vi "MS SQL_InRFID_STN20.vi"(4 "[STATUS]":i32, 6 "RFID":string, 7 "OP10B_002_SLEEVE_PIN_SEAL_ASSY":T1, 8 "error in (no error)":errorcluster, 11 "Ref in":T2={"MS SQL Connection"=refnum, "UDL File"=path "", "Time"="", "DCODE"="", "WIP+1"=0, "MC No?"=0, "POKAYOKE?"=FALSE, "Expected Result"="", "Result [Status]"="", "Clock"=0.0, "RFID"="", "WIP Queue"=refnum, "TS Parameter"={"ProfitCenterCode"="", "LineCode"="", "WorkOrderNumber"="", "Model"="", "Model_with_Prefix"="", "VendorCode"="", "SetParameterDateCode"="", "PokaYoke"=0, "Target"=1, "Live_DateCode"="", "CustomerPartNumber"="", "Hand"="", "Ent_Stamp"=timestamp(0 s since 1904-01-01), "STS_CD"=0.0}, "Data_Queue"=[], "RFID Serial No."=""} {"TS Parameter"."Target" min=1 max=100000; "TS Parameter"."PokaYoke" min=0 max=1}) -> (0 "error out":errorcluster, 2 "Message":picture, 3 "Ref out":T2={"MS SQL Connection"=refnum, "UDL File"=path "", "Time"="", "DCODE"="", "WIP+1"=0, "MC No?"=0, "POKAYOKE?"=FALSE, "Expected Result"="", "Result [Status]"="", "Clock"=0.0, "RFID"="", "WIP Queue"=refnum, "TS Parameter"={"ProfitCenterCode"="", "LineCode"="", "WorkOrderNumber"="", "Model"="", "Model_with_Prefix"="", "VendorCode"="", "SetParameterDateCode"="", "PokaYoke"=0, "Target"=1, "Live_DateCode"="", "CustomerPartNumber"="", "Hand"="", "Ent_Stamp"=timestamp(0 s since 1904-01-01), "STS_CD"=0.0}, "Data_Queue"=[], "RFID Serial No."=""} {"TS Parameter"."Target" min=1 max=100000; "TS Parameter"."PokaYoke" min=0 max=1})   [LabVIEW 2020]
uses:
  Controls/TD SQL.ctl
  <vilib>/addons/database/Connection.llb/Conn ObjectReference.ctl
  Controls/WIP_State.ctl
  Controls/TS_Parameter.ctl
  Controls/OP10B_DataCluster.ctl
  <vilib>/addons/database/NI_Database_API.lvlib
panel:
  out "Query":string
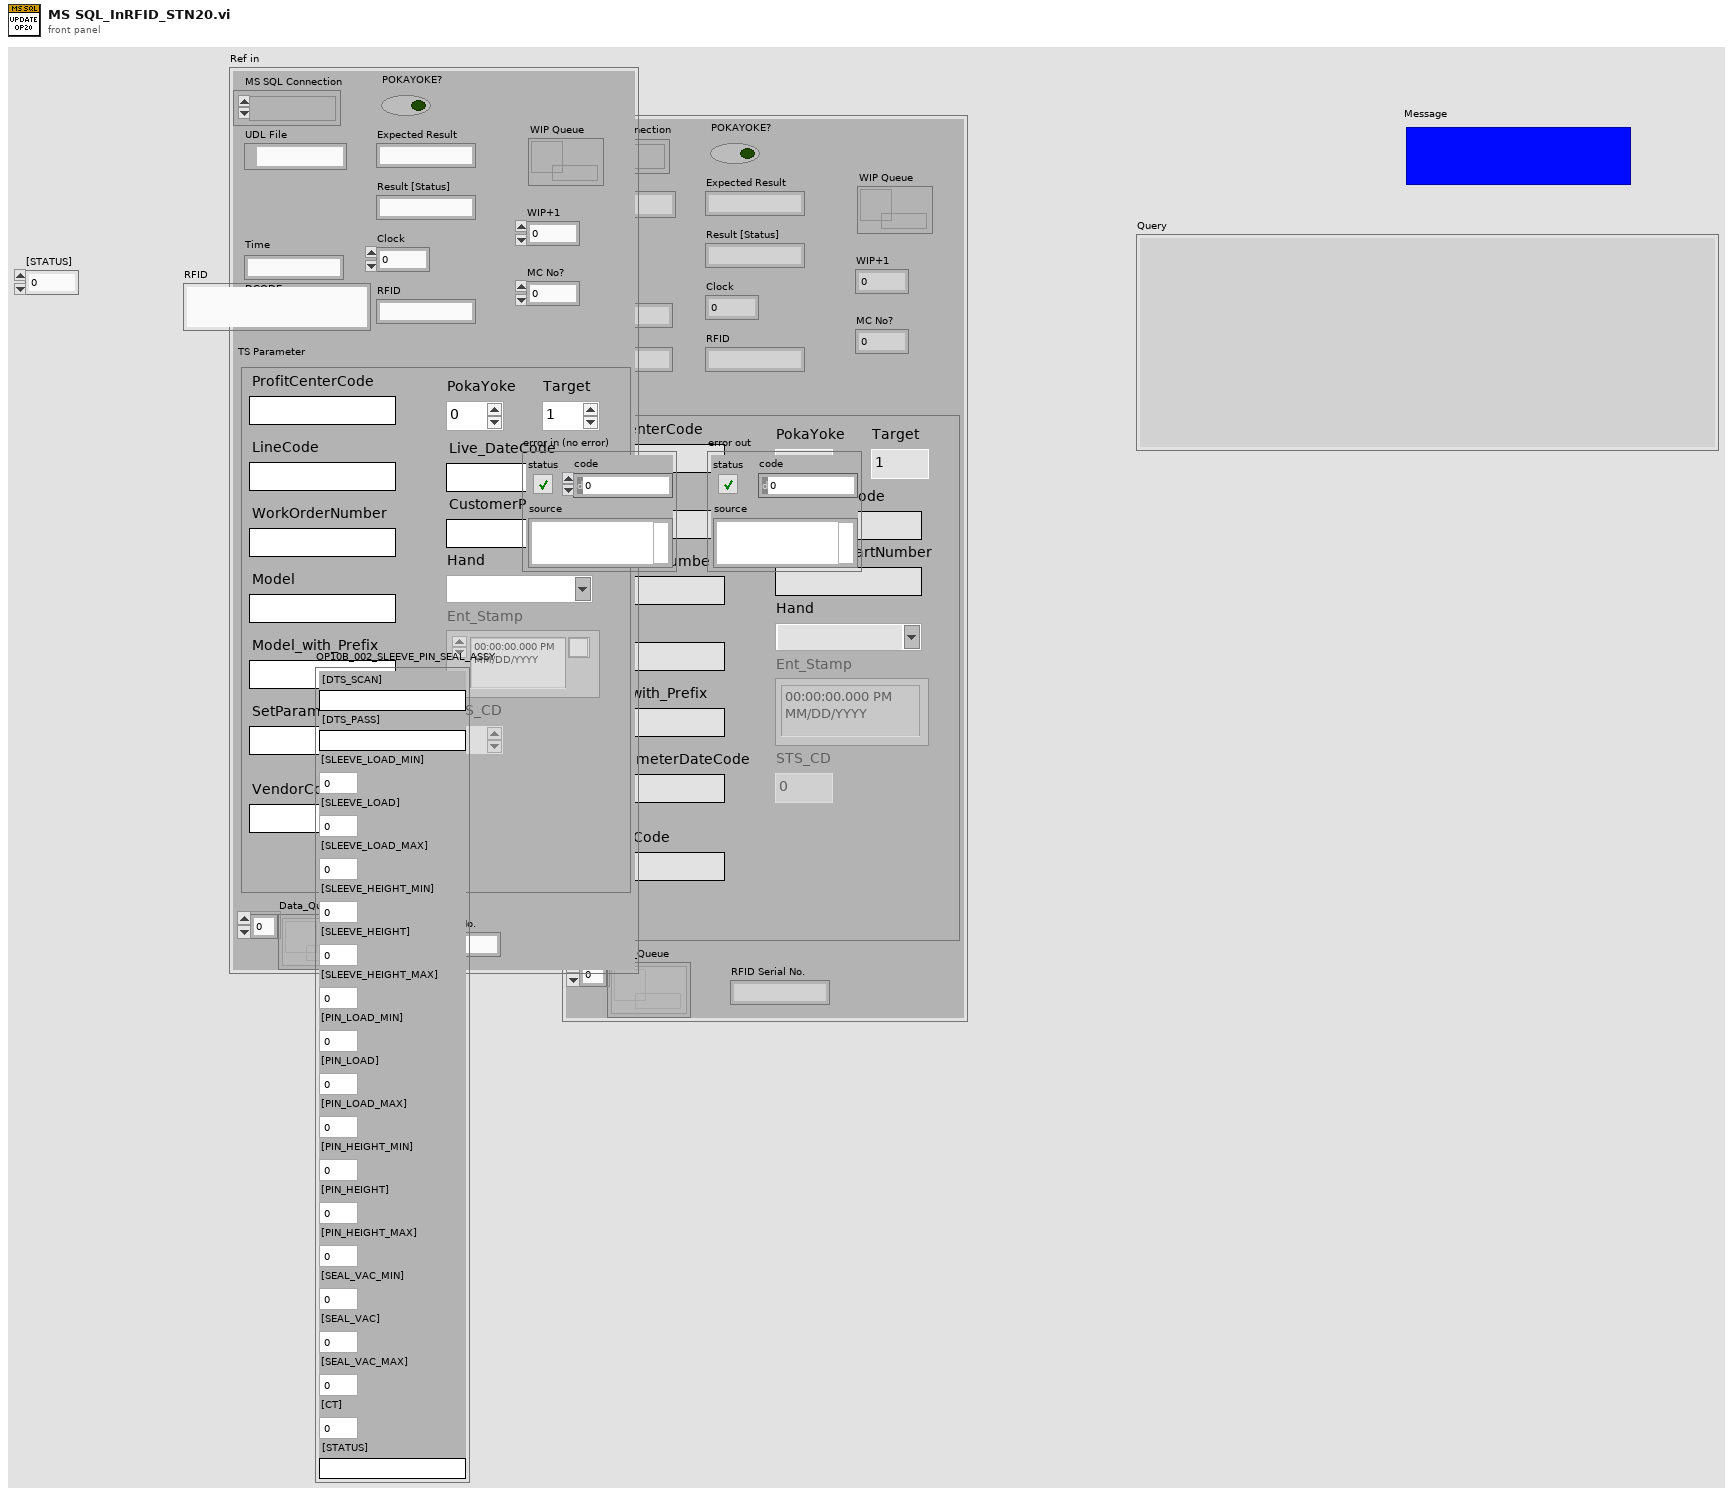
[diagram p1: front panel]
types:
  T1 = typedef "OP10B_DataCluster.ctl" = cluster{"[DTS_SCAN]":string, "[DTS_PASS]":string, "[SLEEVE_LOAD_MIN]":dbl, "[SLEEVE_LOAD]":dbl, "[SLEEVE_LOAD_MAX]":dbl, "[SLEEVE_HEIGHT_MIN]":dbl, "[SLEEVE_HEIGHT]":dbl, "[SLEEVE_HEIGHT_MAX]":dbl, "[PIN_LOAD_MIN]":dbl, "[PIN_LOAD]":dbl, "[PIN_LOAD_MAX]":dbl, "[PIN_HEIGHT_MIN]":dbl, "[PIN_HEIGHT]":dbl, "[PIN_HEIGHT_MAX]":dbl, "[SEAL_VAC_MIN]":dbl, "[SEAL_VAC]":dbl, "[SEAL_VAC_MAX]":dbl, "[CT]":dbl, "[STATUS]":string}
  T2 = typedef "TD SQL.ctl" = cluster{"MS SQL Connection":T3, "UDL File":path, "Time":string, "DCODE":string, "WIP+1":i64, "MC No?":i32, "POKAYOKE?":bool, "Expected Result":string, "Result [Status]":string, "Clock":dbl, "RFID":string, "WIP Queue":refnum<queue>, "TS Parameter":T4, "Data_Queue":refnum<queue>[], "RFID Serial No.":string}
  T3 = typedef "NI_Database_API.lvlib/Conn ObjectReference.ctl" = refnum<k1>
  T4 = typedef "TS_Parameter.ctl" = cluster{"ProfitCenterCode":string, "LineCode":string, "WorkOrderNumber":string, "Model":string, "Model_with_Prefix":string, "VendorCode":string, "SetParameterDateCode":string, "PokaYoke":i32, "Target":i32, "Live_DateCode":string, "CustomerPartNumber":string, "Hand":string, "Ent_Stamp":timestamp, "STS_CD":dbl}
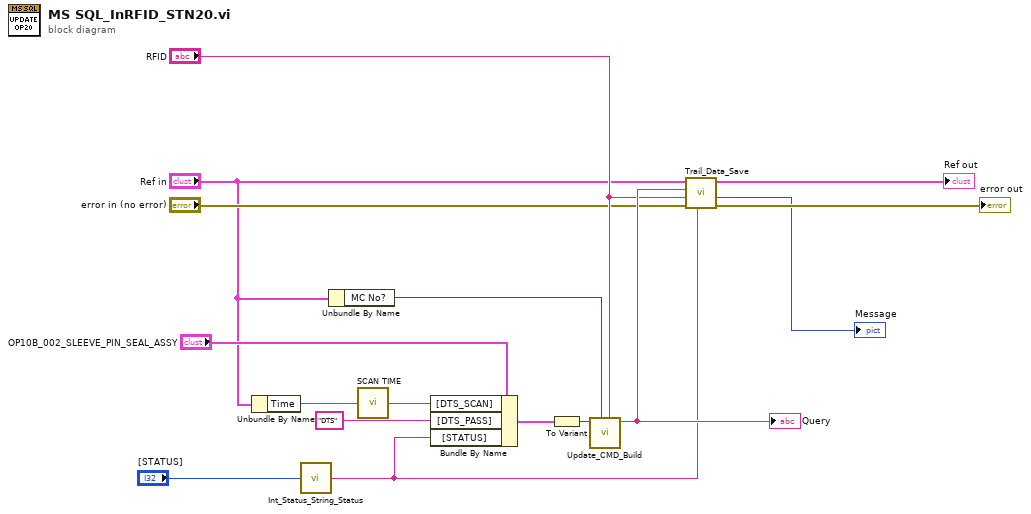
[diagram p0: block diagram]
diagram:
  n1 = Unbundle By Name("Ref in") -> ("Time"=w7:string)
  n2 = call "Int_Status_String_Status.vi"("[STATUS]"="[STATUS]") -> ("STATUS"=w3:string)
  n3 = Unbundle By Name("Ref in") -> ("MC No?"=w1:i32)
  n4 = call "SCAN TIME.vi"("Time in"=w7) -> ("Time out"=w15:string)
  n5 = Bundle By Name(cluster="OP10B_002_SLEEVE_PIN_SEAL_ASSY", "[DTS_SCAN]"=w15, "[DTS_PASS]"="DTS", "[STATUS]"=w3) -> (w16:T1)
  n6 = To Variant(anything=w16) -> (Variant=w12:variant)
  n7 = call "Update_CMD_Build.vi"("RFID"="RFID", "Machine No"=w1, "Variant"=w12) -> ("Update Query"=w11:string)  [unwired: 5 in, 1 out]
  "Query" <- w11
  n8 = call "Trail_Data_Save.vi"("Status"=w3, "error in (no error)"="error in (no error)", "RFID"="RFID", "Query"=w11, "Ref in"="Ref in") -> ("error out"=→"error out":errorcluster, "Message"=→"Message":picture, "Ref Out"=→"Ref out":T2)  [unwired: 1 in, 1 out]
